vi "UpdateACQconf.vi"(8 "error in (no error)":errorcluster, 10 "status":string, 11 "Interface in":refnum<class "Interface.lvclass">) -> (0 "error out":errorcluster, 2 "ACQ conf rx":T1, 3 "Interface out":refnum<class "Interface.lvclass">)   [LabVIEW 2018, in "Interface.lvclass"]
uses:
  Interface.lvclass
panel:
  in  "Acquisition configuration":T1
  in  "Cluster ACQ conf":cluster{"Acquisition configuration":string}
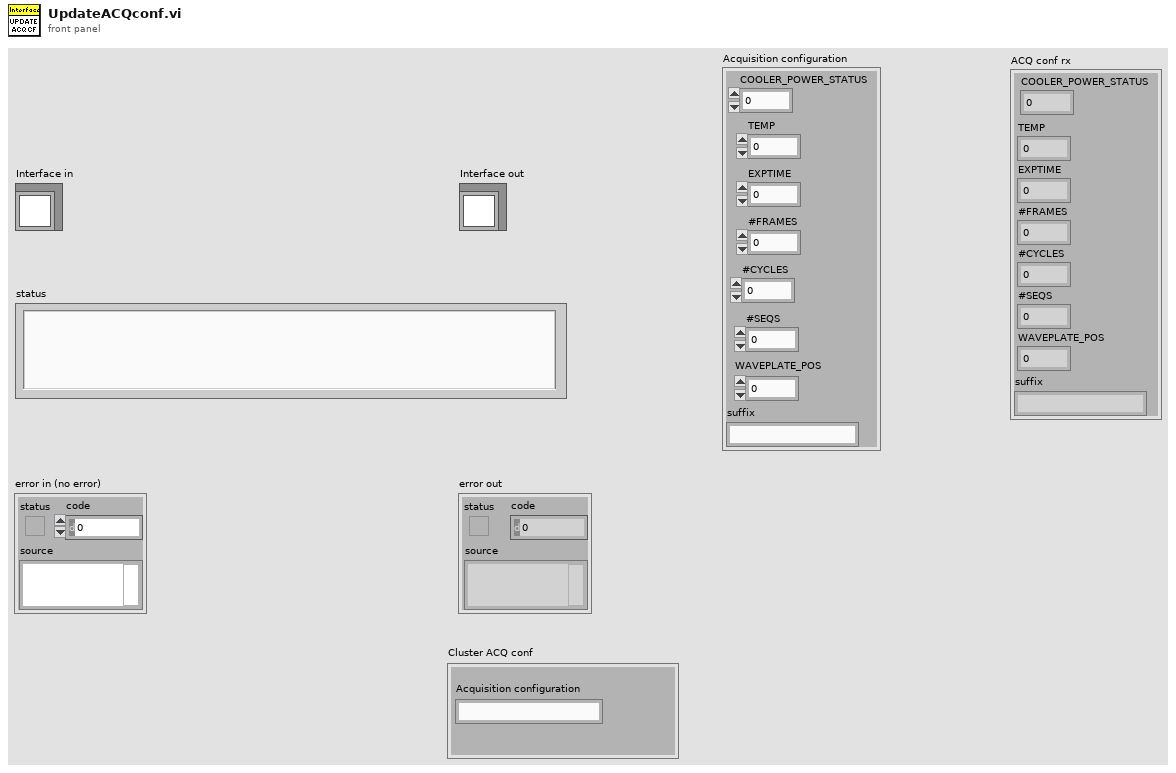
[diagram p1: front panel]
types:
  T1 = cluster{"TEMP":dbl, "EXPTIME":dbl, "#FRAMES":u32, "#CYCLES":u32, "#SEQS":u32, "WAVEPLATE_POS":u32, "COOLER_POWER_STATUS":dbl, "suffix":string}
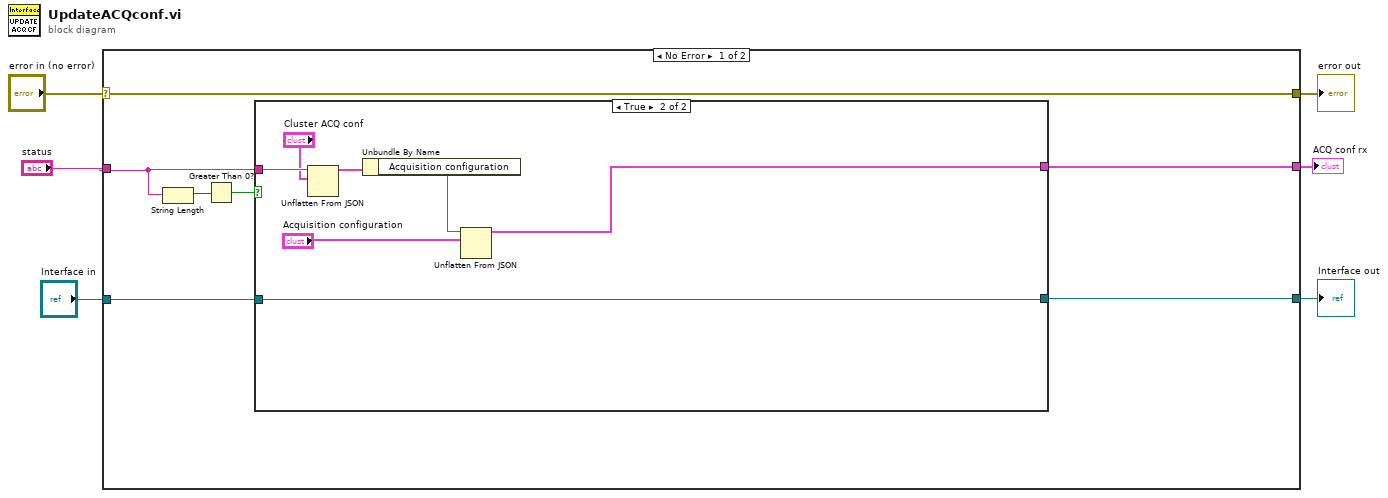
[diagram p0: block diagram]
diagram:
  n1 = case shown="No Error" "error in (no error)" {
    selector: "error in (no error)" -> [w13 w23]
    tunnel: [w13 w23] -> w5
    tunnel: [w12 w22] -> w3
    tunnel: "Interface in" -> [w10 w22]
    tunnel: "status" -> [w8 _]
    tunnel: [w7 _] -> w1
    frame No Error {
      n2 = String Length(string=w8) -> (length=w11:i32)
      n3 = Greater Than 0?(x=w11) -> (x > 0?=w9:bool)
      n4 = case shown="True" w9 {
        tunnel: [w14 w15] -> w12
        tunnel: w8 -> [_ w21]
        tunnel: w10 -> [w14 w15]
        tunnel: [_ w16] -> w7
        frame False {
        }
        frame True {
          n5 = Unflatten From JSON(JSON string=w21, type and defaults="Cluster ACQ conf") -> (value=w19:cluster{"Acquisition configuration":string})  [unwired: 5 in, 1 out]
          n6 = Unbundle By Name(w19) -> ("Acquisition configuration"=w18:string)
          n7 = Unflatten From JSON(JSON string=w18, type and defaults="Acquisition configuration") -> (value=w16:T1)  [unwired: 5 in, 1 out]
        }
      }
    }
    frame Error {
    }
  }
  "error out" <- w5
  "Interface out" <- w3
  "ACQ conf rx" <- w1
